vi "Image colour manipulation.vi"() -> ()   [LabVIEW 2018]
uses:
  Colour Lab Library/VIs/Colour to RGB.vi
  Colour Lab Library/VIs/RGB to Colour.vi
  Colour Lab Library/VIs/RGB Luminosity.vi
  Colour Lab Library/Colour Lab.lvlib
panel:
  out "Inverted image":picture
  out "Greyscaled image":picture
  in  "Input image":picture
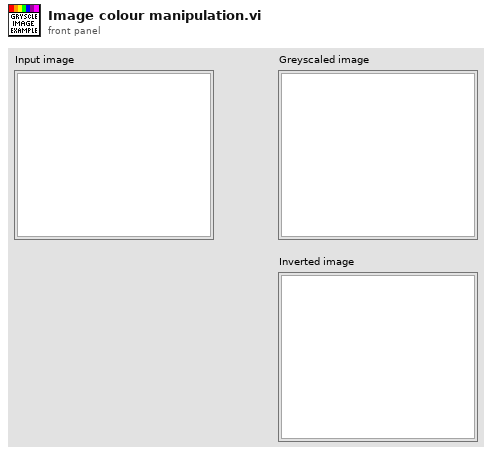
[diagram p1: front panel]
types:
  T1 = typedef "imagedata.ctl" = cluster{"image type":i32, "image depth":i32, "image":u8[], "mask":u8[], "colors":u32[], "Rectangle":cluster{"left":i16, "top":i16, "right":i16, "bottom":i16}}
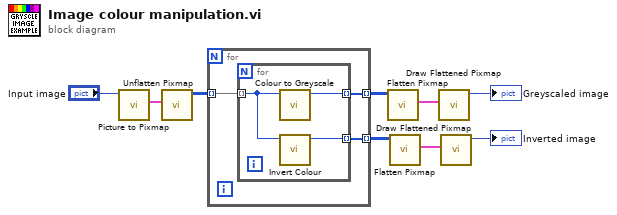
[diagram p0: block diagram]
diagram:
  n1 = call <vilib>:"Picture to Pixmap.vi"("picture"="Input image") -> ("image data"=w9:T1)  [unwired: 9 in, 1 out]
  n2 = call <vilib>:"Unflatten Pixmap.vi"("image data"=w9) -> ("24-bit pixmap"=w7:u32[][])  [unwired: 4 in, 6 out]
  n3 = for {
    tunnel: w7 -> [w12] mode=indexing
    tunnel: [w11] -> w5 mode=indexing
    tunnel: [w10] -> w4 mode=indexing
    n4 = for {
      tunnel: w12 -> [w14] mode=indexing
      tunnel: [w15] -> w11 mode=indexing
      tunnel: [w13] -> w10 mode=indexing
      n5 = call "Colour to Greyscale.vi"("Colour"=w14) -> ("Grey"=w15:u32)  [unwired: 9 in, 1 out]
      n6 = call "Invert Colour.vi"("Colour"=w14) -> ("Inverted Colour"=w13:u32)  [unwired: 9 in, 1 out]
    }
  }
  n7 = call <vilib>:"Flatten Pixmap.vi"("24-bit pixmap"=w5) -> ("image data"=w6:T1)  [unwired: 10 in]
  n8 = call <vilib>:"Flatten Pixmap.vi"("24-bit pixmap"=w4) -> ("image data"=w3:T1)  [unwired: 10 in]
  n9 = call <vilib>:"Draw Flattened Pixmap.vi"("image data"=w6) -> ("new picture"=→"Greyscaled image":picture)  [unwired: 8 in]
  n10 = call <vilib>:"Draw Flattened Pixmap.vi"("image data"=w3) -> ("new picture"=→"Inverted image":picture)  [unwired: 8 in]
